vi "Read Profile from Data File.vi"(0 "Filepath":path, 7 "Controller List":T2(array[cluster]), 11 "Error In":errorcluster) -> (4 "Profile":string[][](array[string]), 6 "Pump Control Style":i32, 8 "TestStyle":string, 10 "VoltLoc":string, 15 "Error Out":errorcluster)   [LabVIEW 2013]
uses:
  TypeDef/Controller Names.ctl
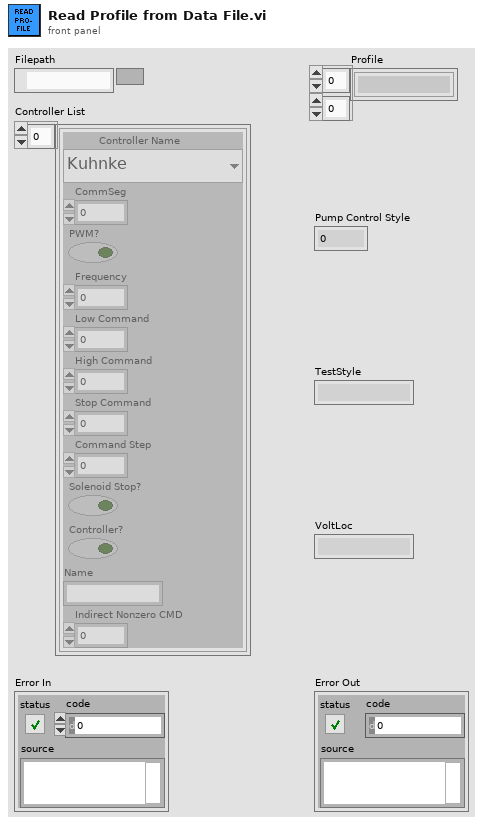
[diagram p1: front panel]
types:
  T1 = typedef "Controller Names.ctl" = enum16{"Kuhnke", "McLaren", "Helbako BLDC", "Conti", "Hella BLDC Screw", "Hella BLDC Turbine", "Helbako (old)", "TI PWM", "PSA", "Hella Gas", "Hella Diesel", "8 Comm", "10 Comm", "8 Comm Hella", "10 Comm Hella", "8 Comm Omron", "10 Comm Omron", "8 Comm Nissan", "10 Comm Nissan"}
  T2 = cluster{"Controller Name":T1, "CommSeg":i32, "PWM?":bool, "Frequency":i32, "Low Command":dbl, "High Command":dbl, "Stop Command":dbl, "Command Step":dbl, "Solenoid Stop?":bool, "Controller?":bool, "Name":string, "Indirect Nonzero CMD":dbl}[]
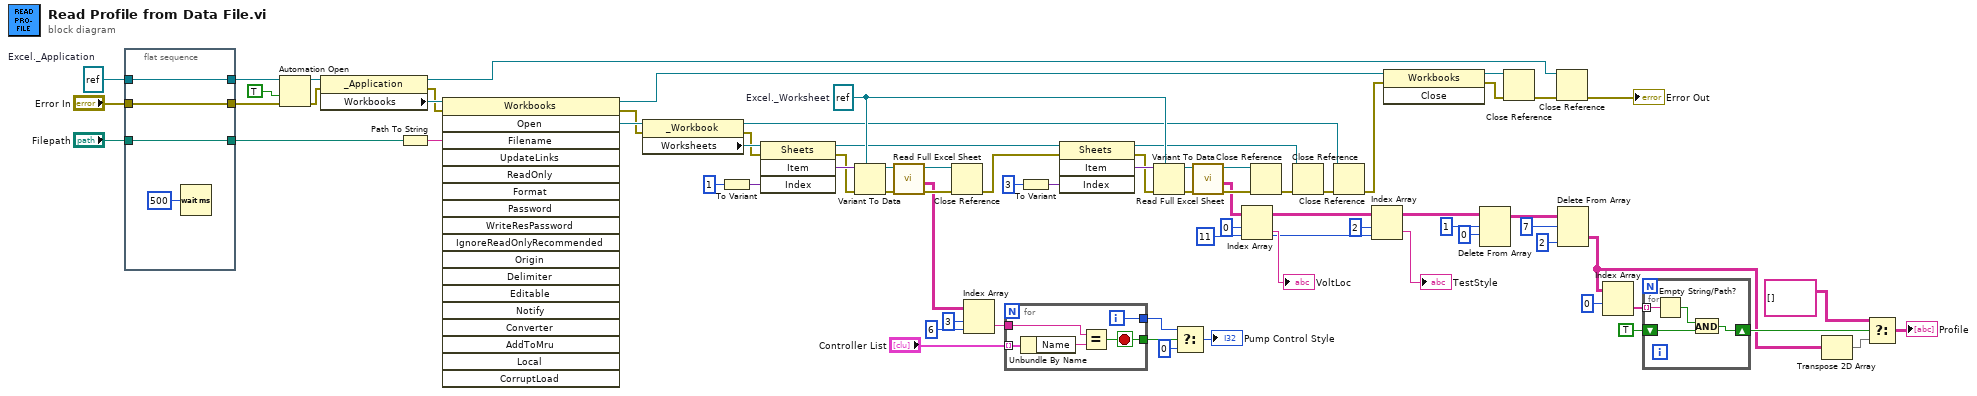
[diagram p0: block diagram]
diagram:
  w14 = 11 ("disabled index (col)")
  w59 = refnum<k7> refnum  # Excel._Worksheet
  w45 = refnum<k7> refnum  # Excel._Application
  n1 = flat-sequence {
    tunnel: w45 -> [w76]
    tunnel: "Error In" -> [w77]
    tunnel: "Filepath" -> [w78]
    tunnel: [w78] -> w43
    tunnel: [w77] -> w42
    tunnel: [w76] -> w41
    frame #0 {
      n2 = Wait (ms)(milliseconds to wait=u32 500) -> ()  [unwired: 1 out]
    }
  }
  n3 = Automation Open(error in (no error)=w42, Automation Refnum=w41, 9:TRUE ("open new instance (false)")) -> (Automation Refnum=w72:refnum<k7>, error out=w73:errorcluster)  [unwired: 1 in]
  n4 = property class="_Application"(reference=w72, error in=w73) -> (reference out=w52:refnum<k7>, error out=w71:errorcluster, "Workbooks"=w74:refnum<k7>)
  n5 = Path To String(path=w43) -> (string=w70:string)
  n6 = invoke class="Workbooks" method="Open"(reference=w74, error in=w71, "Filename"=w70) -> (reference out=w50:refnum<k7>, error out=w53:errorcluster, "Open"=w54:refnum<k7>)  [unwired: 15 in, 15 out]
  n7 = property class="_Workbook"(reference=w54, error in=w53) -> (reference out=w55:refnum<k7>, error out=w67:errorcluster, "Worksheets"=w68:refnum<k7>)
  n8 = To Variant(anything=1) -> (Variant=w66:variant)
  n9 = invoke class="Sheets" method="Item"(reference=w68, error in=w67, "Index"=w66) -> (reference out=w11:refnum<k7>, error out=w64:errorcluster, "Item"=w65:variant)  [unwired: 1 in, 1 out]
  n10 = Variant To Data(error in=w64, type=w59, Variant=w65) -> (data=w62:refnum<k7>, error out=w63:errorcluster)
  n11 = call "Read Full Excel Sheet.vi"("Error In"=w63, "Excel._Worksheet"=w62) -> ("Error Out"=w61:errorcluster, "Data"=w9:string[][], "Reference Out"=w60:refnum<k7>)  [unwired: 7 in]
  n12 = Close Reference(reference=w60, error in (no error)=w61) -> (error out=w10:errorcluster)
  n13 = Index Array(array=w9, index (row)=3, index (col)=6 ("disabled index (col)")) -> (element=w6:string)
  n14 = for {
    tunnel: w6 -> [w83]
    tunnel: "Controller List" -> [w79] mode=indexing
    tunnel: [w81] -> w2
    tunnel: [w80] -> w3
    i -> [w81]
    stop <- w80 stop-if-true
    n15 = Unbundle By Name(w79) -> ("Name"=w82:string)
    n16 = Equal?(x=w83, y=w82) -> (x = y?=w80:bool)
  }
  n17 = To Variant(anything=3) -> (Variant=w39:variant)
  n18 = invoke class="Sheets" method="Item"(reference=w11, error in=w10, "Index"=w39) -> (reference out=w56:refnum<k7>, error out=w37:errorcluster, "Item"=w38:variant)  [unwired: 1 in, 1 out]
  n19 = Variant To Data(error in=w37, type=w59, Variant=w38) -> (data=w35:refnum<k7>, error out=w36:errorcluster)
  n20 = Select(t=w2, s=w3, f=0) -> (s? t:f=→"Pump Control Style":i32)
  n21 = call "Read Full Excel Sheet.vi"("Error In"=w36, "Excel._Worksheet"=w35) -> ("Error Out"=w34:errorcluster, "Data"=w15:string[][], "Reference Out"=w33:refnum<k7>)  [unwired: 7 in]
  n22 = Index Array(array=w15, index (row)=0, index (col)=w14) -> (element=→"VoltLoc":string)
  n23 = Close Reference(reference=w33, error in (no error)=w34) -> (error out=w58:errorcluster)
  n24 = Close Reference(reference=w56, error in (no error)=w58) -> (error out=w57:errorcluster)
  n25 = Close Reference(reference=w55, error in (no error)=w57) -> (error out=w48:errorcluster)
  n26 = Index Array(array=w15, index (row)=2, index (col)=w14) -> (element=→"TestStyle":string)
  n27 = invoke class="Workbooks" method="Close"(reference=w50, error in=w48) -> (reference out=w46:refnum<k7>, error out=w47:errorcluster)  [unwired: 1 in, 1 out]
  n28 = Delete From Array(array=w15, length=1, index (row)=0) -> (array with subset deleted=w29:string[][])  [unwired: 1 in, 1 out]
  n29 = Close Reference(reference=w46, error in (no error)=w47) -> (error out=w49:errorcluster)
  n30 = Close Reference(reference=w52, error in (no error)=w49) -> (error out=→"Error Out":errorcluster)
  n31 = Delete From Array(array=w29, length=7, index (col)=2 ("disabled index (col)")) -> (deleted portion=w16:string[][])  [unwired: 1 in, 1 out]
  n32 = Index Array(array=w16, index (row)=0) -> (element=w26:string[])  [unwired: 1 in]
  n33 = for {
    tunnel: w26 -> [w87] mode=indexing
    shift-right: [w85] -> w23
    shift-left: TRUE -> [w84]
    n34 = Empty String/Path?(string/path=w87) -> (empty?=w86:bool)
    n35 = And(x=w86, y=w84) -> (x .and. y?=w85:bool)
  }
  n36 = Transpose 2D Array(2D array=w16) -> (transposed array=w21:string[][])
  n37 = Select(t=string[][] [], s=w23, f=w21) -> (s? t:f=→"Profile":string[][])
